vi "PositionOpen WO Configuration.vi"(8 "DeviceStatus":errorcluster, 11 "PositionSensorIndex":T2) -> (0 "error out":errorcluster)   [LabVIEW 2014]
uses:
  <vilib>/Rock Robotics/SystemInterfaces/Encoder/FPGA_EncoderIdx.ctl
  <vilib>/Rock Robotics/SystemInterfaces/Position/PositionDevRef.ctl
panel:
  out "PositionSensor Reference":T1
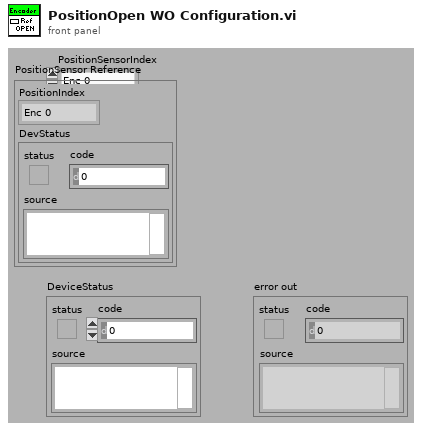
[diagram p1: front panel]
types:
  T1 = typedef "PositionDevRef.ctl" = cluster{"PositionIndex":T2, "DevStatus":errorcluster}
  T2 = typedef "FPGA_EncoderIdx.ctl" = enum8{"Enc 0", "Enc 1", "Enc 2", "Enc 3", "Enc 4", "Enc 5", "Enc 6", "Enc 7", "Invalid"}
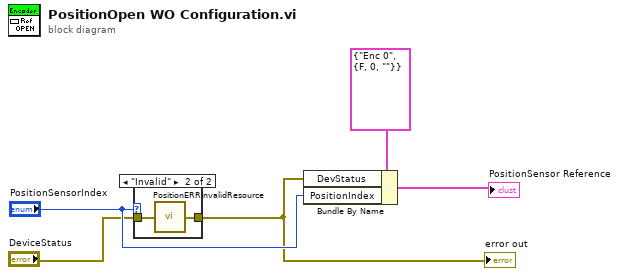
[diagram p0: block diagram]
diagram:
  n1 = case shown="\"Invalid\"" "PositionSensorIndex" {
    tunnel: [w6 w8] -> w3
    tunnel: "DeviceStatus" -> [w6 w7]
    frame Default {
    }
    frame "Invalid" {
      n2 = call "PositionERRInvalidResource.vi"("error in (no error)"=w7) -> ("error out"=w8:errorcluster)
    }
  }
  "error out" <- w3
  n3 = Bundle By Name(cluster=T1 {"PositionIndex"=enum."Enc 0", "DevStatus"={"status"=FALSE, "code"=0, "source"=""}} ("Encoder Reference out"), "DevStatus"=w3, "PositionIndex"="PositionSensorIndex") -> (→"PositionSensor Reference":T1)
